vi "Position Check.vi"(8 "data value reference 2":refnum<data-value>, 11 "data value reference":refnum<data-value>) -> (0 "Y-Offset":dbl, 1 "X-Offset":dbl, 2 "XY Graph":T1(graph))   [LabVIEW 2021]
uses:
  State Estimator/Measurements.ctl
  IMU/IMU Data.ctl
  Steering Motor Encoder/Steering Motor Encoder Data.ctl
  GNSS/GNSS Data.ctl
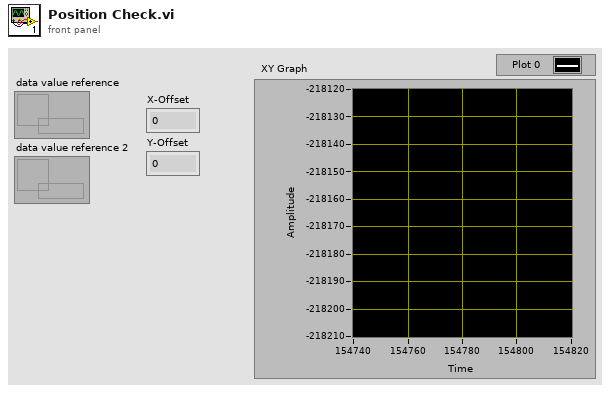
[diagram p1: front panel]
types:
  T1 = cluster{"Trajectory(X/Y/PSI)":dbl[], "Trajectory(X/Y/PSI)":dbl[]}
  T2 = typedef "Measurements.ctl" = cluster{"IMU Data":T3, "Steering Motor Encoder Data":T4, "GNSS Data":T5}
  T3 = typedef "IMU Data.ctl" = cluster{"Gyroscope":cluster{"X (rad/s)":dbl, "Y (rad/s)":dbl, "Z (rad/s)":dbl}, "Accelerometer":cluster{"X (m/s^2)":dbl, "Y (m/s^2)":dbl, "Z (m/s^2)":dbl}, "Flag IMU":dbl}
  T4 = typedef "Steering Motor Encoder Data.ctl" = cluster{"Encoder Position (counts)":i32, "Steering Angle (rad)":dbl, "Steering Encoder Iteration":dbl}
  T5 = typedef "GNSS Data.ctl" = cluster{"Latitude (rad)":dbl, "Longitude (rad)":dbl, "Altitude (m)":dbl, "Speed (m/s)":dbl, "Heading (rad)":dbl, "Fix Quality":i32, "Number of Satellites":i32, "Latitude (deg)":dbl, "Longitude (deg)":dbl, "Flag GNSS":dbl}
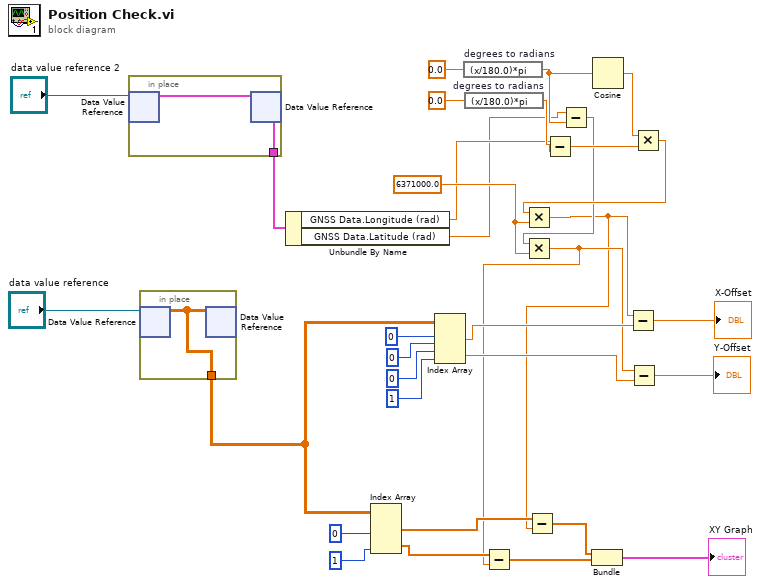
[diagram p0: block diagram]
diagram:
  w20 = 6371000.0
  n1 = in-place {
    in-place-border: [w33] -> w28
    n2 = in-place-dvr #1("data value reference 2") -> (w33:T2)  [unwired: 1 out]
    n3 = in-place-dvr #1(w33) -> ()  [unwired: 2 out]
  }
  n4 = in-place {
    in-place-border: [w34] -> w23
    n5 = in-place-dvr #2("data value reference") -> (w34:dbl[][])  [unwired: 1 out]
    n6 = in-place-dvr #2(w34) -> ()  [unwired: 2 out]
  }
  n7 = Unbundle By Name(w28) -> ("GNSS Data.Longitude (rad)"=w13:dbl, "GNSS Data.Latitude (rad)"=w12:dbl)
  n8 = Index Array(array=w23, index (col) #1=0, index (col) #2=1) -> (element #1=w6:dbl[], element #2=w7:dbl[])  [unwired: 2 in]
  n9 = Index Array(array=w23, index (row) #1=0, index (col) #1=0, index (row) #2=0, index (col) #2=1) -> (element #1=w9:dbl, element #2=w8:dbl)
  n10 = expression code="(x/180.0)*pi" "degrees to radians"(0.0 ("y")) -> (w16:dbl)
  n11 = expression code="(x/180.0)*pi" "degrees to radians"(0.0 ("y")) -> (w17:dbl)
  n12 = Subtract(x=w13, y=w17) -> (x-y=w14:dbl)
  n13 = Subtract(x=w12, y=w16) -> (x-y=w10:dbl)
  n14 = Multiply(x=w10, y=w20) -> (x*y=w2:dbl)
  n15 = Subtract(x=w7, y=w2) -> (x-y=w4:dbl[])
  n16 = Cosine(x=w16) -> (cos(x)=w15:dbl)
  n17 = Subtract(x=w2, y=w8) -> (x-y=→"Y-Offset":dbl)
  n18 = Multiply(x=w15, y=w14) -> (x*y=w11:dbl)
  n19 = Multiply(x=w11, y=w20) -> (x*y=w1:dbl)
  n20 = Subtract(x=w6, y=w1) -> (x-y=w5:dbl[])
  n21 = Bundle(w5, w4) -> (→"XY Graph":cluster{dbl[], dbl[]})  [unwired: 1 in]
  n22 = Subtract(x=w1, y=w9) -> (x-y=→"X-Offset":dbl)
